vi "F Dwf Get Last Error.vi"(8 "error in (no error)":errorcluster, 11 "pdwferc":i32) -> (0 "error out":errorcluster, 2 "function return":i32, 3 "pdwferc out":i32)   [LabVIEW 2019, in "Olasdwf.lvlib"]
doc: "DWFAPI int FDwfGetLastError(DWFERC *pdwferc);"
uses:
  Olasdwf.lvlib
  Windows/System32/dwf.dll
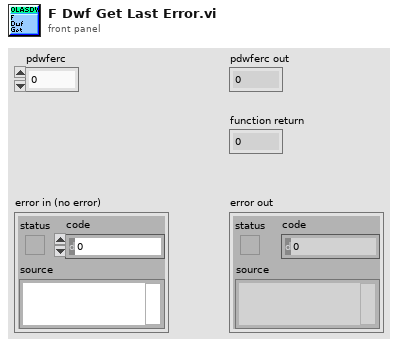
[diagram p1: front panel]
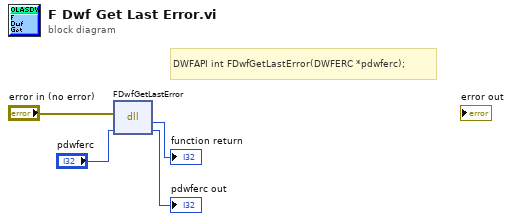
[diagram p0: block diagram]
diagram:
  # "DWFAPI int FDwfGetLastError(DWFERC *pdwferc);"
  n1 = dll-call lib="C:/Windows/System32/dwf.*" fn="FDwfGetLastError"(error in="error in (no error)", "pdwferc"="pdwferc") -> (→"function return":i32, "pdwferc"=→"pdwferc out":i32)  [unwired: 2 in, 2 out]
